vi "Pattern Matching.vi"() -> ()   [LabVIEW 2016]
doc: "This example shows how to use the color pattern matching tools in NI Vision.\n\nYou use color pattern matching to locate known reference or fiducial patterns in an image quickly. Pattern matching is the key to many applications. Color pattern matching can provide your application with information about the presence or absence, number, and location of the model within an image.\n\nYou use color pattern matching in the following three general applications areas:\n\n* Alignment -- Determine the position and orientation of a known object by locating features. You use the features as points of reference on the object.\n\n* Gauging -- Measure lengths, diameters, angles, and other critical dimensions. If the measurements fall outside of set tolerance levels, the component is rejected. You sometimes use gauging in-line with the manufacturing process and off-line. If you make the measurements off-line, a sample of components is used to determine the quality of a lot or batch of manufactured components.\n\n* Inspection -- Detect simple flaws, such as missing parts or unreadable printing."
uses:
  <vilib>/vision/NI_Vision_Development_Module.lvlib
panel:
  out "Number of Matches":i32
  out "Results":T1(array[cluster]) {"Score" format="%.1f"; "Position"."Y" format="%.2g"; "Position"."X" format="%.2g"}
  in  "Max # of Matches":i32=5
  in  "Minimum Score":sgl=700.0
  out "Template":T2(plugin-control)
  in  "Stop":bool
  out "Image":T2(plugin-control)
  # "Overview: Demonstrates how to perform Pattern Matching using two steps that include learning the pattern template defined by a Region of Interest (ROI) and then matching the learned template in the image.\nRequirements: Vision Development Software.\nInstructions:\n1. Run the VI.\n2. Draw a ROI in the image to define the template. The learned template is displayed in the Template display and the match results are overlaid on the Image display."
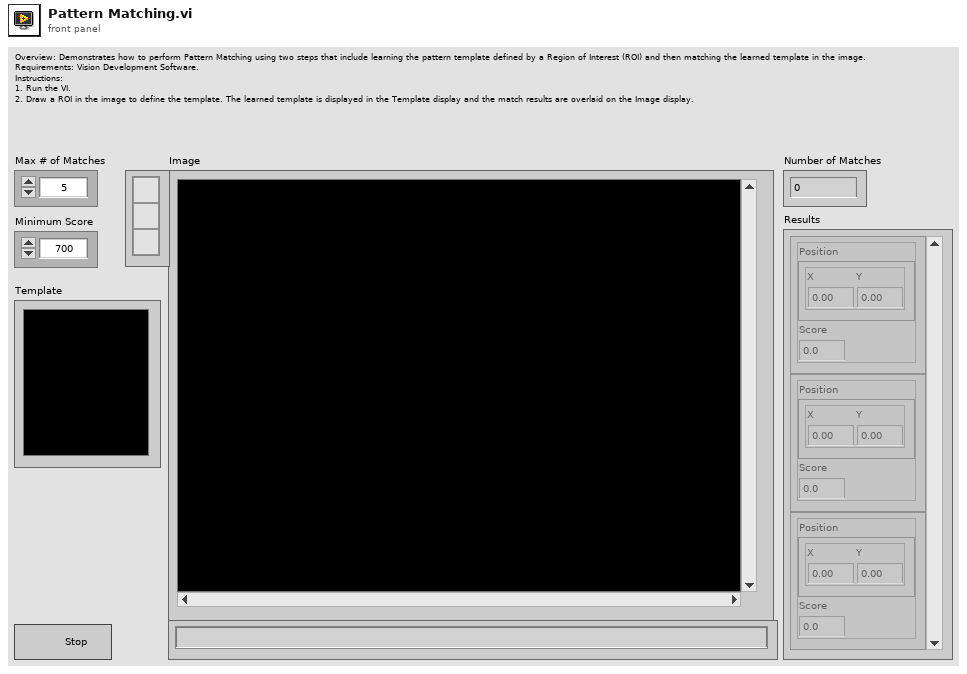
[diagram p1: front panel]
types:
  T1 = cluster{"Position":cluster{"X":dbl, "Y":dbl}, "Score":sgl}[]
  T2 = typedef "IMAQ Image.ctl" = refnum<image>
  T3 = typedef "Image Type" = u32
  T4 = typedef "IMAQ Rectangle" = cluster{"Left":i32, "Top":i32, "Right":i32, "Bottom":i32, "Rotation":dbl}
  T5 = typedef "ROI Descriptor" = cluster{"Global Rectangle":i32[], "Contours":cluster{"ID":enum32{"External", "Internal"}, "Type":u32, "Coordinates":i32[]}[]}
  T6 = cluster{"Max # of Matches":i32, "Minimum Score":sgl}
  T7 = cluster{"Max # of Matches":i32, "Minimum Score":sgl, "Angle Ranges":cluster{"Start Angle":sgl, "End Angle":sgl}[]}
  T8 = cluster{"Position":cluster{"x":sgl, "y":sgl}, "Angle":sgl, "Scale":sgl, "Score":sgl, "Bounding Box":cluster{"x":sgl, "y":sgl}[]}[]
  T9 = cluster{"Position":cluster{"x":sgl, "y":sgl}, "Score":sgl}
  T10 = cluster{i32[], cluster{"Contour Type":u32, "ROI Type":u32, i32[]}[]}
  T11 = cluster{"Global Rectangle":i32[], "Contours":cluster{"Contour Type":u32, "ROI Type":u32, "Points":i32[]}[]}
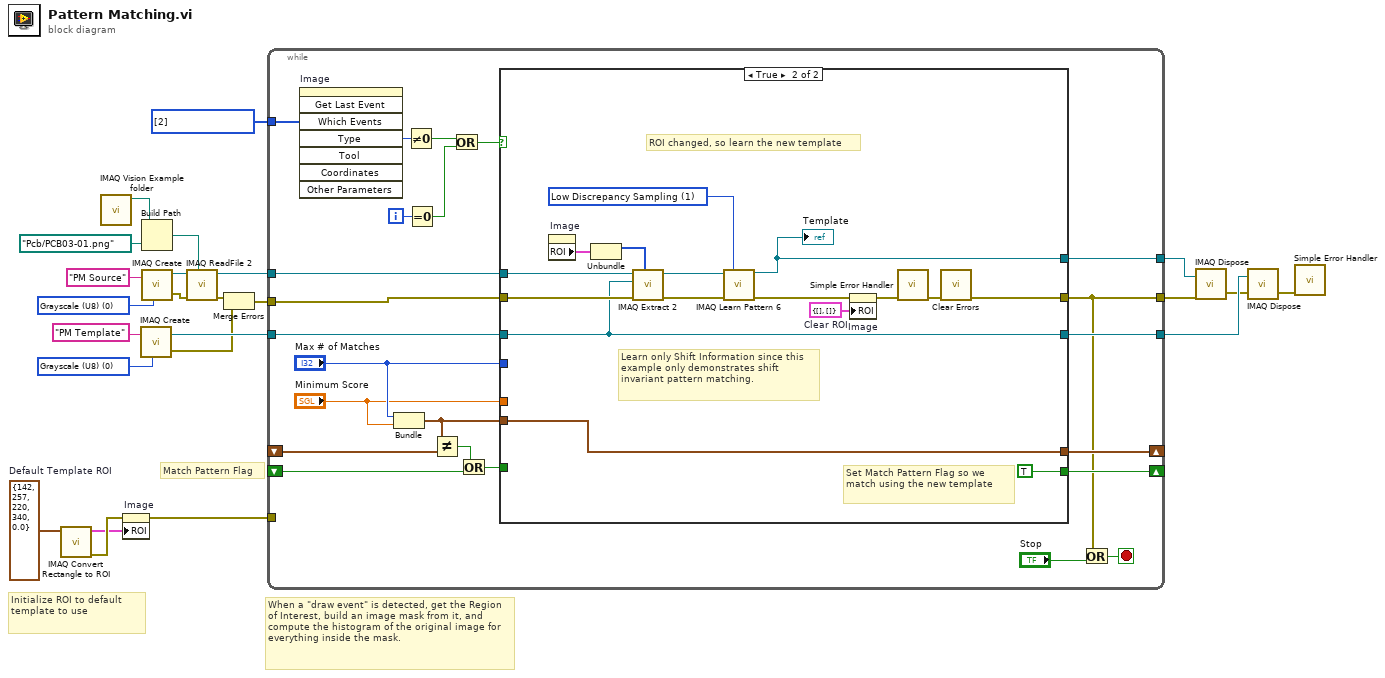
[diagram p0: block diagram]
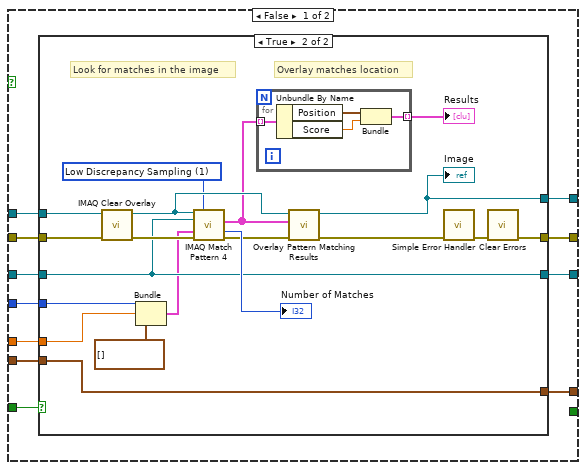
[diagram p2: hidden frame]
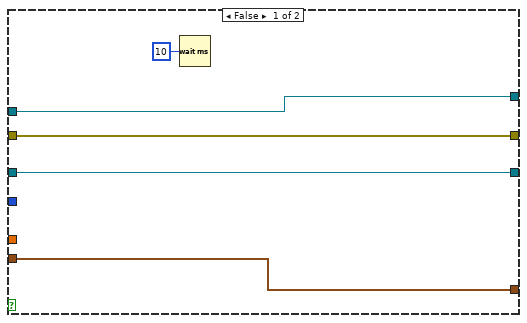
[diagram p3: hidden frame]
diagram:
  w12 = T3 0 items=["Grayscale (U8)", "Grayscale (I16)", "Grayscale (SGL)", "Complex (CSG)", "RGB (U32)", "HSL (U32)", "RGB (U64)", "Grayscale (U16)"] ("Image Type")
  w13 = T3 0 items=["Grayscale (U8)", "Grayscale (I16)", "Grayscale (SGL)", "Complex (CSG)", "RGB (U32)", "HSL (U32)", "RGB (U64)", "Grayscale (U16)"] ("Image Type")
  w18 = i32[] [2] items=["No Event"=0, "Click Event"=1, "Draw Event"=2, "Size Event"=4, "Scroll Event"=5, "Double Click Event"=8] ("Which Events")
  w20 = T4 {"Left"=142, "Top"=257, "Right"=220, "Bottom"=340, "Rotation"=0.0}  # Default Template ROI
  # "Initialize ROI to default template to use"
  # "When a \"draw event\" is detected, get the Region of Interest, build an image mask from it, and compute the histogram of the original image for everything inside the mask."
  # "Match Pattern Flag"
  n1 = call "IMAQ Convert Rectangle to ROI"("Rectangle"=w20) -> ("error out"=w8:errorcluster, "ROI Descriptor"=w2:T5)  [unwired: 8 in]
  n2 = call "IMAQ Vision Example folder.vi"() -> ("Example Image Path"=w23:path)  [unwired: 11 in]
  n3 = property on="Image" class="ImageControl"(error in=w8, "ROI"=w2) -> (error out=w1:errorcluster)  [unwired: 1 in, 1 out]
  n4 = call "IMAQ Create"("Image Name"="PM Template", "Image Type"=w12) -> ("New Image"=w17:T2, "error out"=w6:errorcluster)  [unwired: 3 in]
  n5 = Build Path(base path=w23, name or relative path=path "Pcb/PCB03-01.png") -> (appended path=w19:path)
  n6 = call "IMAQ Create"("Image Name"="PM Source", "Image Type"=w13) -> ("New Image"=w4:T2, "error out"=w9:errorcluster)  [unwired: 3 in]
  n7 = call "IMAQ ReadFile 2"("File Path"=w19, "error in (no error)"=w9, "Image"=w4) -> ("error out"=w7:errorcluster, "Image Out"=w3:T2)  [unwired: 4 in, 3 out]
  n8 = Merge Errors(w7, w6) -> (w5:errorcluster)
  n9 = while {
    tunnel: w3 -> [w37]
    tunnel: w18 -> [w47]
    tunnel: w17 -> [w36]
    tunnel: w5 -> [w41]
    shift-right: [w35] -> _
    shift-left: _ -> [w29]
    shift-right: [w40] -> _
    shift-left: _ -> [w39]
    tunnel: [w33] -> w16
    tunnel: [w34] -> w15
    tunnel: [w27] -> w14
    tunnel: w1 -> [_]
    i -> [w44]
    stop <- w25 stop-if-true
    n10 = invoke on="Image" class="ImageControl" method="Get Last Event"("Which Events"=w47) -> ("Type"=w46:i32)  [unwired: 7 in, 7 out]
    n11 = Bundle("Max # of Matches"="Max # of Matches", "Minimum Score"="Minimum Score") -> (w30:T6)  [unwired: 1 in]
    n12 = Not Equal To 0?(x=w46) -> (x != 0?=w45:bool)
    n13 = Equal To 0?(x=w44) -> (x = 0?=w43:bool)
    n14 = Not Equal?(x=w30, y=w29) -> (x != y?=w28:bool)
    n15 = Or(x=w45, y=w43) -> (x .or. y?=w42:bool)
    n16 = Or(x=w28, y=w39) -> (x .or. y?=w38:bool)
    n17 = case shown="True" w42 {
      tunnel: w37 -> [w56 w97]
      tunnel: w41 -> [w55 w96]
      tunnel: w36 -> [w54 w90]
      tunnel: [_ TRUE] -> w40
      tunnel: w38 -> [w58 _]
      tunnel: w30 -> [w57 w89]
      tunnel: [w53 w93] -> w27
      tunnel: [w52 w89] -> w35
      tunnel: [w51 w90] -> w34
      tunnel: [w50 w91] -> w33
      tunnel: "Max # of Matches" -> [w49 _]
      tunnel: "Minimum Score" -> [w48 _]
      frame False {
        n18 = case shown="True" w58 {
          tunnel: w57 -> [w61 w80]
          tunnel: w56 -> [w59 w82]
          tunnel: w55 -> [w63 w81]
          tunnel: w54 -> [w60 w74]
          tunnel: [w63 w78] -> w53
          tunnel: [w61 w80] -> w52
          tunnel: [w60 w74] -> w51
          tunnel: [w59 w73] -> w50
          tunnel: w49 -> [_ w68]
          tunnel: w48 -> [_ w67]
          frame False {
            n19 = Wait (ms)(milliseconds to wait=u32 10) -> ()  [unwired: 1 out]
          }
          frame True {
            w64 = 1 items=["All", "Low Discrepancy Sampling", "Grayscale Value Pyramid", "Gradients Pyramid"] ("Algorithm")
            # "Overlay matches location"
            # "Look for matches in the image"
            n20 = call "IMAQ Clear Overlay"("error in (no error)"=w81, "Image"=w82) -> ("error out"=w77:errorcluster, "Image Out"=w71:T2)  [unwired: 8 in]
            n21 = Bundle("Max # of Matches"=w68, "Minimum Score"=w67, "Angle Ranges"=cluster{"Start Angle":sgl, "End Angle":sgl}[] []) -> (w66:T7)  [unwired: 1 in]
            n22 = call "IMAQ Match Pattern 4"("Image"=w71, "Algorithm"=w64, "Template Image"=w74, "Parameters"=w66, "error in (no error)"=w77) -> ("Matches (pixel)"=w70:T8, "Number of Matches"=→"Number of Matches":i32, "error out"=w69:errorcluster)  [unwired: 6 in, 2 out]
            n23 = for {
              tunnel: w70 -> [w86] mode=indexing
              tunnel: [w83] -> w76 mode=indexing
              n24 = Unbundle By Name(w86) -> ("Position"=w85:cluster{"x":sgl, "y":sgl}, "Score"=w84:sgl)
              n25 = Bundle("Position"=w85, "Score"=w84) -> (w83:T9)  [unwired: 1 in]
            }
            "Results" <- w76
            n26 = call "Overlay Pattern Matching Results.vi"("error in"=w69, "Matches"=w70, "Image"=w71) -> ("error out"=w72:errorcluster, "Image Out"=w73:T2)  [unwired: 7 in]
            "Image" <- w73
            n27 = call <vilib>:"Simple Error Handler.vi"("error in (no error)"=w72) -> ("error out"=w79:errorcluster)  [unwired: 4 in, 4 out]
            n28 = call <vilib>:"Clear Errors.vi"("error in (no error)"=w79) -> ("error out"=w78:errorcluster)  [unwired: 5 in, 1 out]
          }
        }
      }
      frame True {
        w87 = 1 items=["All", "Low Discrepancy Sampling", "Grayscale Value Pyramid", "Gradients Pyramid"] ("Algorithm")
        w98 = T10 {[], []}  # Clear ROI
        # "Set Match Pattern Flag so we match using the new template"
        # "Learn only Shift Information since this example only demonstrates shift invariant pattern matching."
        # "ROI changed, so learn the new template"
        n29 = property on="Image" class="ImageControl"() -> ("ROI"=w100:T11)  [unwired: 2 in, 2 out]
        n30 = Unbundle(w100) -> ("Global Rectangle"=w102:i32[])  [unwired: 1 out]
        n31 = call "IMAQ Extract 2"("Optional Rectangle"=w102, "error in (no error)"=w96, "Image Dst"=w90, "Image Src"=w97) -> ("error out"=w88:errorcluster, "Image Dst Out"=w101:T2)  [unwired: 6 in]
        n32 = call "IMAQ Learn Pattern 6"("Image"=w101, "Algorithm"=w87, "error in (no error)"=w88) -> ("Template Image Out"=w91:T2, "error out"=w92:errorcluster)  [unwired: 10 in, 1 out]
        "Template" <- w91
        n33 = property on="Image" class="ImageControl"(error in=w92, "ROI"=w98) -> (error out=w99:errorcluster)  [unwired: 1 in, 1 out]
        n34 = call <vilib>:"Simple Error Handler.vi"("error in (no error)"=w99) -> ("error out"=w94:errorcluster)  [unwired: 4 in, 4 out]
        n35 = call <vilib>:"Clear Errors.vi"("error in (no error)"=w94) -> ("error out"=w93:errorcluster)  [unwired: 5 in, 1 out]
      }
    }
    n36 = Or(x=w27, y="Stop") -> (x .or. y?=w25:bool)
  }
  n37 = call "IMAQ Dispose"("Image"=w16, "error in (no error)"=w14) -> ("error out"=w11:errorcluster)  [unwired: 4 in]
  n38 = call "IMAQ Dispose"("Image"=w15, "error in (no error)"=w11) -> ("error out"=w10:errorcluster)  [unwired: 4 in]
  n39 = call <vilib>:"Simple Error Handler.vi"("error in (no error)"=w10) -> ()  [unwired: 4 in, 5 out]
